vi "Inst_CNT90.vi"(8 "error in":errorcluster, 10 "All Message Queues in":T1, 11 "Prueba21_1 in":refnum<class "Prueba21.lvclass">) -> (0 "error out":errorcluster)   [LabVIEW 2019, in "Prueba21.lvclass"]
uses:
  Prueba21.lvclass
  QMH/Message Queue/All Message Queues.ctl
  QMH/Message Queue/Message Cluster.ctl
  Prueba21.lvclass/Prueba21.ctl
  <vilib>/Utility/error.llb/Error Cluster From Error Code.vi
  QMH/Message Queue/Enqueue Message (Single).vi
  <vilib>/ErrorRing/Error Ring.xnode
  QMH/Message Queue/Message Queue.lvlib
  Instrumento/CNT90/CNT90.lvclass
panel:
  out "All States":string[](array[string])
  out "Actual State":string
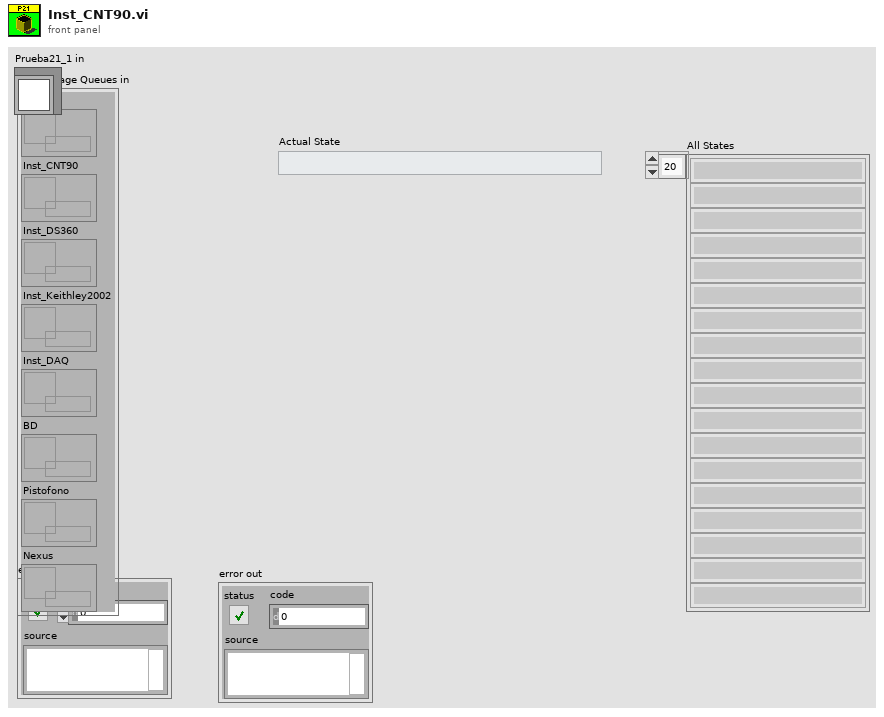
[diagram p1: front panel]
types:
  T1 = typedef "Message Queue.lvlib/All Message Queues.ctl" = cluster{"MHL":refnum<queue>, "Inst_CNT90":refnum<queue>, "Inst_DS360":refnum<queue>, "Inst_Keithley2002":refnum<queue>, "Inst_DAQ":refnum<queue>, "BD":refnum<queue>, "Pistofono":refnum<queue>, "Nexus":refnum<queue>}
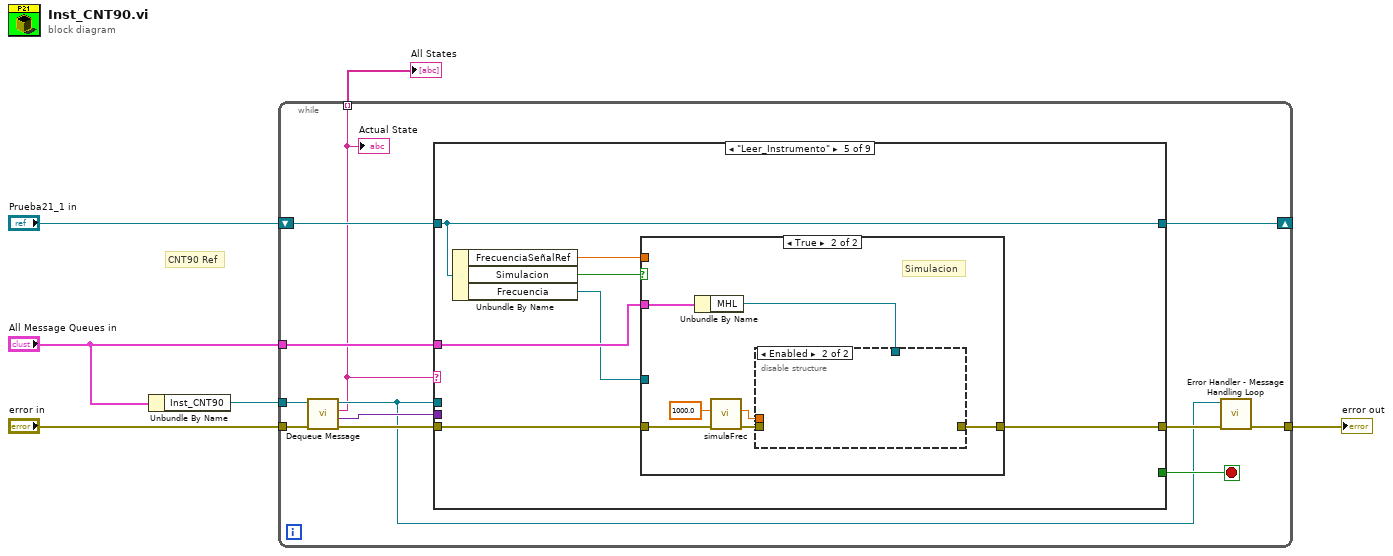
[diagram p0: block diagram]
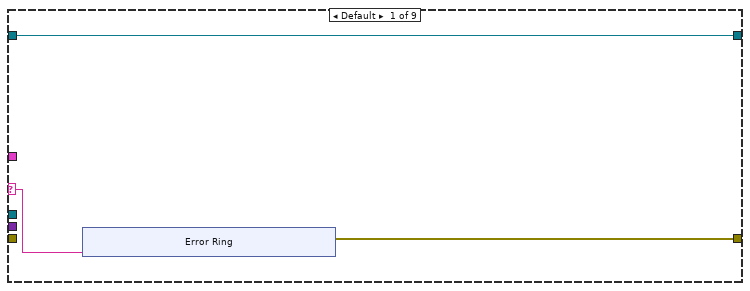
[diagram p2: hidden frame]
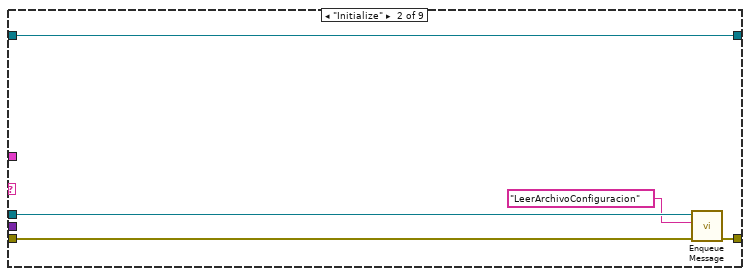
[diagram p3: hidden frame]
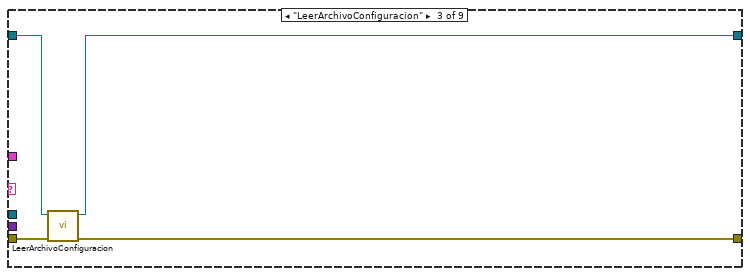
[diagram p4: hidden frame]
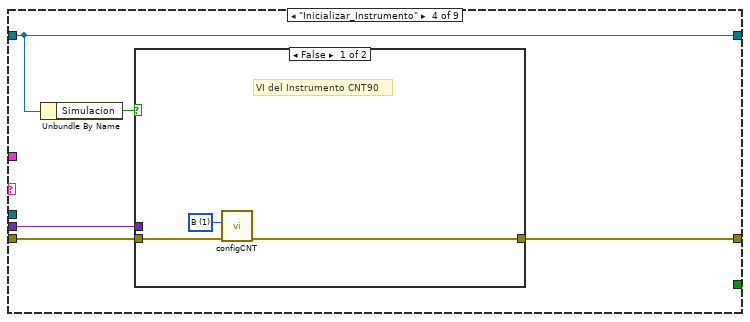
[diagram p5: hidden frame]
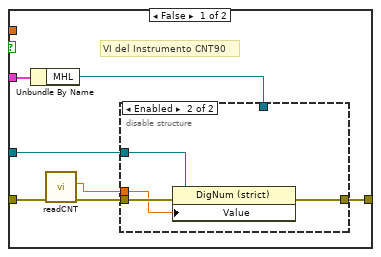
[diagram p7: hidden frame]
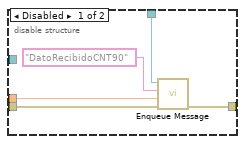
[diagram p8: hidden frame]
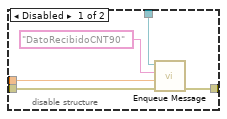
[diagram p9: hidden frame]
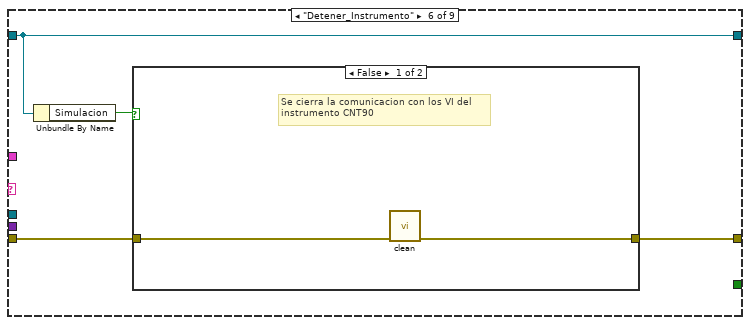
[diagram p10: hidden frame]
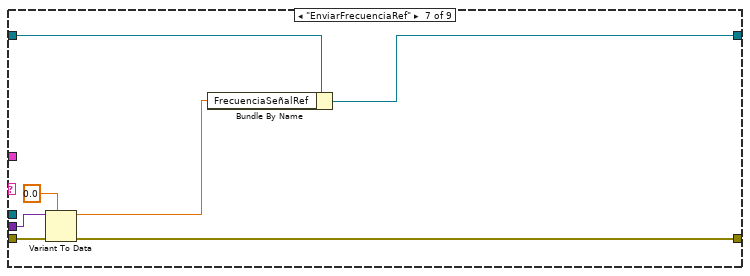
[diagram p12: hidden frame]
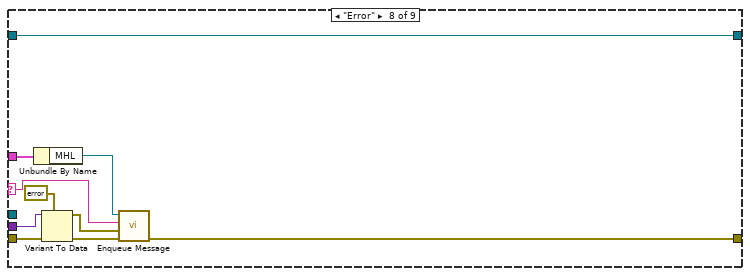
[diagram p13: hidden frame]
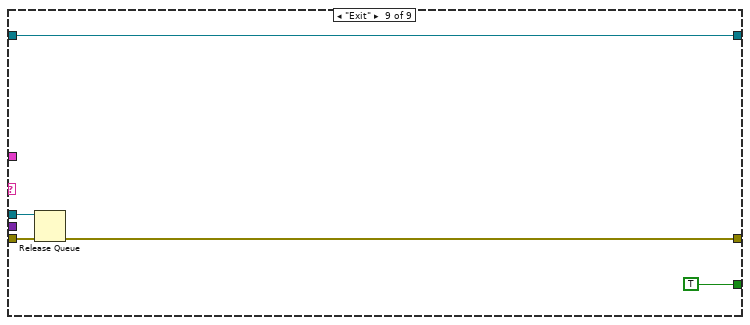
[diagram p14: hidden frame]
diagram:
  # "CNT90 Ref"
  n1 = Unbundle By Name("All Message Queues in") -> ("Inst_CNT90"=w4:refnum<queue>)
  n2 = while {
    tunnel: "error in" -> [w18]
    tunnel: w4 -> [w17]
    tunnel: "All Message Queues in" -> [w16]
    tunnel: [w9] -> w2
    shift-right: [w12] -> _
    shift-left: "Prueba21_1 in" -> [w15]
    tunnel: [w7] -> w1 mode=indexing
    stop <- w11 stop-if-true
    n3 = call "Dequeue Message.vi"("error in (no error)"=w18, "Message Queue"=w17) -> ("error out"=w13:errorcluster, "Message Data"=w14:variant, "Message"=w7:string, "dup Message Queue"=w8:refnum<queue>)  [unwired: 6 in]
    "Actual State" <- w7
    n4 = case shown="\"Leer_Instrumento\"" w7 {
      selector: w7 -> [w21 _ _ _ _ _ _ w100 _]
      tunnel: w16 -> [_ _ _ _ w50 _ _ w99 _]
      tunnel: w15 -> [w19 w33 w35 w42 w52 w84 w90 w97 w107]
      tunnel: w8 -> [_ w30 _ _ _ _ _ _ w109]
      tunnel: w14 -> [_ _ _ w38 _ _ w93 w103 _]
      tunnel: w13 -> [_ w31 w37 w41 w53 w82 w94 w104 w110]
      tunnel: [w20 w32 w34 w39 w48 w85 w95 w96 w106] -> w10
      tunnel: [w19 w33 w36 w42 w52 w84 w91 w97 w107] -> w12
      tunnel: [_ _ _ _ _ _ _ _ TRUE] -> w11
      frame Default {
        n5 = xnode "Error Ring"("parameter 0"=w21) -> ("error out"=w20:errorcluster)
      }
      frame "Initialize" {
        n6 = call-poly "Enqueue Message.vi"("error in (no error)"=w31, "Message"="LeerArchivoConfiguracion", "Message Queue"=w30) -> ("error out"=w32:errorcluster)  [unwired: 7 in, 1 out]
      }
      frame "LeerArchivoConfiguracion" {
        n7 = call "LeerArchivoConfiguracion.vi"("error in"=w37, "Prueba31 in"=w35) -> ("error out"=w34:errorcluster, "Prueba31 out"=w36:refnum<class "Prueba21.lvclass">)  [unwired: 8 in]
      }
      frame "Inicializar_Instrumento" {
        n8 = Unbundle By Name(w42) -> ("Simulacion"=w40:bool)
        n9 = case shown="False" w40 {
          tunnel: [w45 w46] -> w39
          tunnel: w41 -> [w44 w46]
          tunnel: w38 -> [_ _]
          frame False {
            w43 = 1 items=["A", "B"] ("Channel  1")
            # "VI del Instrumento CNT90"
            n10 = call "configCNT.vi"("error in (no error)"=w44, "Channel  1"=w43) -> ("error out"=w45:errorcluster)  [unwired: 8 in, 1 out]
          }
          frame True {
            # "Simulacion"
          }
        }
      }
      frame "Leer_Instrumento" {
        n11 = Unbundle By Name(w52) -> ("FrecuenciaSeñalRef"=w49:dbl, "Simulacion"=w51:bool, "Frecuencia"=w47:refnum<vi>)
        n12 = case shown="True" w51 {
          tunnel: [w58 w76] -> w48
          tunnel: w53 -> [w60 w73]
          tunnel: w50 -> [w57 w75]
          tunnel: w49 -> [_ _]
          tunnel: w47 -> [w54 _]
          frame False {
            # "VI del Instrumento CNT90"
            n13 = Unbundle By Name(w57) -> ("MHL"=w56:refnum<queue>)
            n14 = call "readCNT.vi"("error in (no error)"=w60) -> ("error out"=w59:errorcluster, "medicion"=w55:dbl)  [unwired: 8 in, 1 out]
            n15 = disable-structure shown="Enabled" {
              disable-tunnel: w59 -> [w64 w69]
              disable-tunnel: [w63 w68] -> w58
              disable-tunnel: w56 -> [w62 _]
              disable-tunnel: w55 -> [w61 w66]
              disable-tunnel: w54 -> [_ w67]
              frame Disabled {
                n16 = call-poly "Enqueue Message.vi"("error in (no error)"=w64, "Message Data"=w61, "Message"="DatoRecibidoCNT90", "Message Queue"=w62) -> ("error out"=w63:errorcluster)  [unwired: 6 in, 1 out]
              }
              frame Enabled {
                n17 = property class="DigNum (strict)"(reference=w67, error in=w69, "Value"=w66) -> (error out=w68:errorcluster)  [unwired: 1 out]
              }
            }
          }
          frame True {
            # "Simulacion"
            n18 = Unbundle By Name(w75) -> ("MHL"=w74:refnum<queue>)
            n19 = call "simulaFrec.vi"("error in (no error)"=w73, "frec in"=1000.0) -> ("error out"=w72:errorcluster, "frec out"=w71:dbl)  [unwired: 7 in, 1 out]
            n20 = disable-structure shown="Enabled" {
              disable-tunnel: [w80 _] -> w76
              disable-tunnel: w74 -> [w79 _]
              disable-tunnel: w72 -> [w78 _]
              disable-tunnel: w71 -> [w77 _]
              frame Disabled {
                n21 = call-poly "Enqueue Message.vi"("error in (no error)"=w78, "Message Data"=w77, "Message"="DatoRecibidoCNT90", "Message Queue"=w79) -> ("error out"=w80:errorcluster)  [unwired: 6 in, 1 out]
              }
              frame Enabled {
              }
            }
          }
        }
      }
      frame "Detener_Instrumento" {
        n22 = Unbundle By Name(w84) -> ("Simulacion"=w83:bool)
        n23 = case shown="False" w83 {
          tunnel: [w87 w88] -> w85
          tunnel: w82 -> [w86 w88]
          frame False {
            # "Se cierra la comunicacion con los VI del\ninstrumento CNT90"
            n24 = call "clean.vi"("error in (no error)"=w86) -> ("error out"=w87:errorcluster)  [unwired: 9 in, 1 out]
          }
          frame True {
            # "Simulacion"
          }
        }
      }
      frame "EnviarFrecuenciaRef" {
        n25 = Variant To Data(error in=w94, type=0.0, Variant=w93) -> (data=w89:dbl, error out=w95:errorcluster)
        n26 = Bundle By Name(cluster=w90, "FrecuenciaSeñalRef"=w89) -> (w91:refnum<class "Prueba21.lvclass">)
      }
      frame "Error" {
        n27 = Unbundle By Name(w99) -> ("MHL"=w98:refnum<queue>)
        n28 = Variant To Data(error in=w104, type=errorcluster {"status"=FALSE, "code"=0, "source"=""} ("error constant"), Variant=w103) -> (data=w101:errorcluster, error out=w102:errorcluster)
        n29 = call-poly "Enqueue Message.vi"("error in (no error)"=w102, "Message Data"=w101, "Message"=w100, "Message Queue"=w98) -> ("error out"=w96:errorcluster)  [unwired: 6 in, 1 out]
      }
      frame "Exit" {
        n30 = Release Queue(queue=w109, error in (no error)=w110) -> (error out=w106:errorcluster)  [unwired: 1 in, 2 out]
      }
    }
    n31 = call "Error Handler - Message Handling Loop.vi"("error in (no error)"=w10, "Message Queue"=w8) -> ("dup error in"=w9:errorcluster)  [unwired: 8 in, 1 out]
  }
  "error out" <- w2
  "All States" <- w1
